vi "NI6071E.contents.vi"   [LabVIEW 2014, in "NI6071E.lvlib"]
doc: "This class is forseen to measure the current of the pulsed power of PHELIX. It interacts with a DAQ card in an NI PXI Chasis.\n\nThis class is part of the PHELIX device layer."
uses:
  NI6071E.lvlib
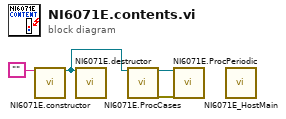
[diagram p0: block diagram]
diagram:
  n1 = call "NI6071E.constructor.vi"("name"="") -> ("i ref out"=w1:refnum<vi>)  [unwired: 16 in, 2 out]
  n2 = call "NI6071E.destructor.vi"("i ref in"=w1) -> ()  [unwired: 18 in, 1 out]
  n3 = call "NI6071E.ProcCases.vi"("i ref in"=w1) -> ("i ref out"=w3:refnum<vi>, "error out"=w2:errorcluster)  [unwired: 16 in, 1 out]
  n4 = call "NI6071E.ProcPeriodic.vi"("i ref in"=w3, "error in (no error)"=w2) -> ()  [unwired: 15 in, 3 out]
  n5 = call "NI6071E_HostMain.vi"() -> ()  [unwired: 1 in]
